vi "Init.vi"(10 "input":string[](array[string]), 11 "Volcano in":refnum<class "Volcano.lvclass">) -> (3 "Volcano out":refnum<class "Volcano.lvclass">)   [LabVIEW 2023, in "d16.lvlib" / "Volcano.lvclass"]
uses:
  Volcano.lvclass
  Volcano.lvclass/Volcano.ctl
  317e8209-662c-4c31-af41-99644d260e76.vi
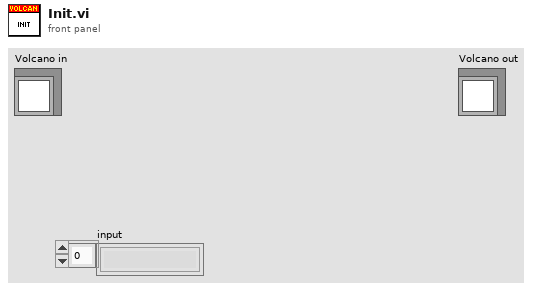
[diagram p1: front panel]
types:
  T1 = map{string, cluster{"Flow Rate":i32, "Routes":string[], "Route Time":i32[]}}
  T2 = cluster{"Current Valve":string, "Unopened Valves":string[], "Cumulative Pressure Released":u64, "Time":i32}
  T3 = cluster{"Flow Rate":i32, "Routes":string[], "Route Time":i32[]}
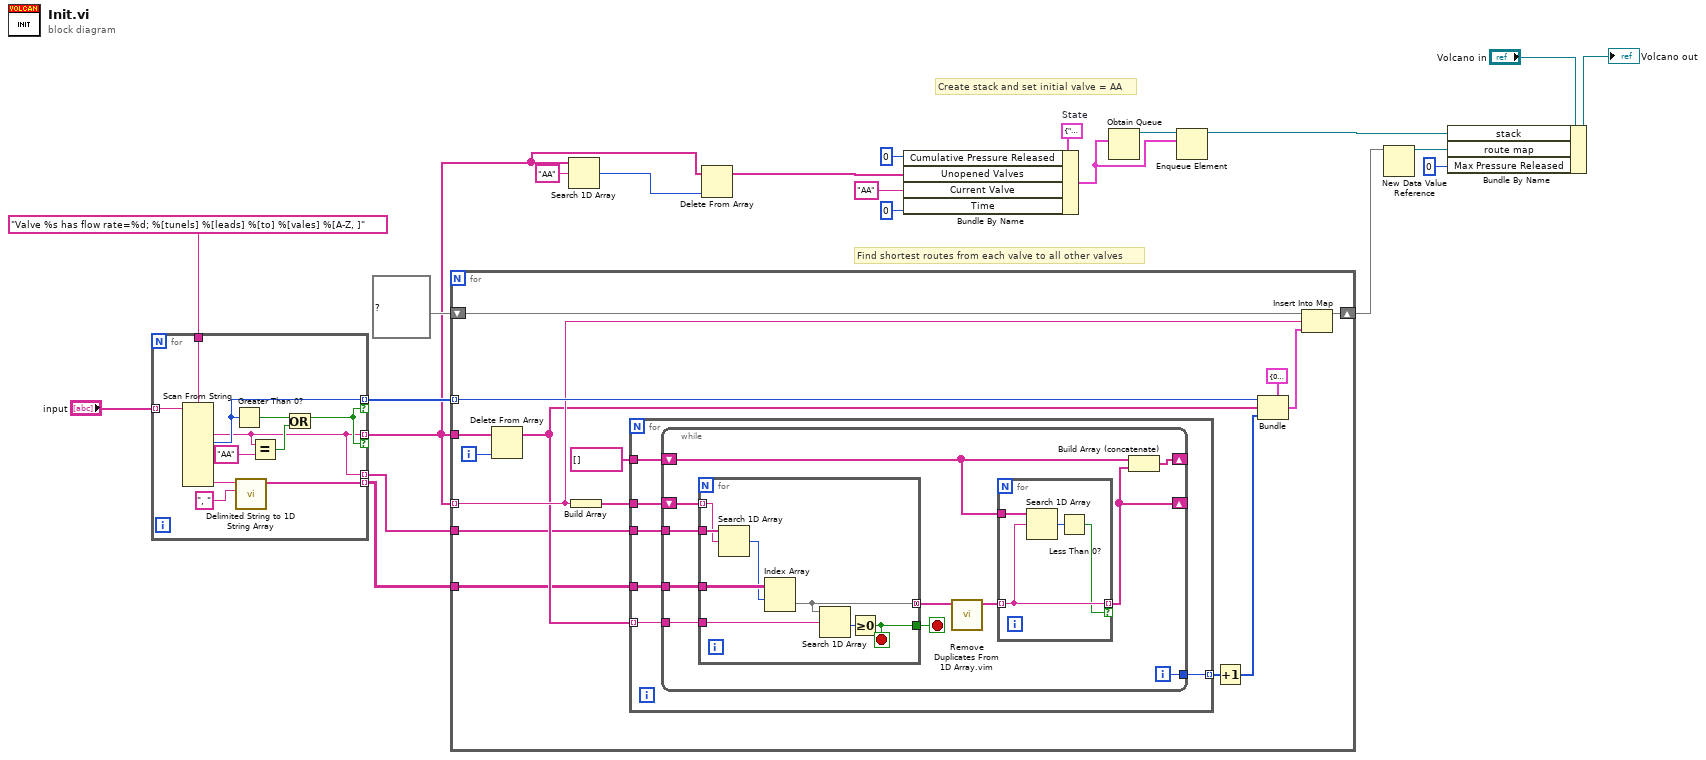
[diagram p0: block diagram]
diagram:
  w15 = T2 {"Current Valve"="AA", "Unopened Valves"=["AA"], "Cumulative Pressure Released"=0, "Time"=0}  # State
  # "Find shortest routes from each valve to all other valves"
  # "Create stack and set initial valve = AA"
  n1 = for {
    tunnel: "input" -> [w33] mode=indexing
    tunnel: "Valve %s has flow rate=%d; %[tunels] %[leads] %[to] %[vales] %[A-Z, ]" ("format string") -> [w32]
    tunnel: [w24] -> w2 mode=indexing if=w26
    tunnel: [w24] -> w20 mode=indexing
    tunnel: [w29] -> w19 mode=indexing if=w26
    tunnel: [w27] -> w18 mode=indexing
    n2 = Scan From String(format string=w32, input string=w33) -> (output 1=w24:string, output 2=w29:i32, output 7=w30:string)  [unwired: 13 in, 3 out]
    n3 = Greater Than 0?(x=w29) -> (x > 0?=w28:bool)
    n4 = call <vilib>:"Delimited String to 1D String Array.vi"("delimiter"=", ", "delimited string"=w30) -> ("string array"=w27:string[])  [unwired: 9 in]
    n5 = Equal?(x=w24, y="AA") -> (x = y?=w25:bool)
    n6 = Or(x=w28, y=w25) -> (x .or. y?=w26:bool)
  }
  n7 = for {
    tunnel: w20 -> [w40]
    tunnel: w2 -> [w42] mode=indexing
    tunnel: w2 -> [w46]
    shift-right: [w48] -> w7
    shift-left: T1 {} ("map out") -> [w47]
    tunnel: w19 -> [w44] mode=indexing
    tunnel: w18 -> [w39]
    i -> [w45]
    n8 = Delete From Array(array=w46, index=w45) -> (array with subset deleted=w41:string[])  [unwired: 1 in, 1 out]
    n9 = Build Array(w42) -> (w38:string[])
    n10 = for {
      tunnel: w41 -> [w54] mode=indexing
      tunnel: w40 -> [w53]
      tunnel: w39 -> [w52]
      tunnel: w38 -> [w51]
      tunnel: [w50] -> w37 mode=indexing
      tunnel: string[] [] -> [w49]
      n11 = while {
        tunnel: w54 -> [w63]
        tunnel: w53 -> [w65]
        shift-right: [w55] -> _
        shift-left: w51 -> [w60]
        tunnel: [w62] -> w50
        shift-right: [w56] -> _
        shift-left: w49 -> [w57]
        tunnel: w52 -> [w64]
        i -> [w62]
        stop <- w61 stop-if-true
        n12 = for {
          tunnel: w65 -> [w77]
          tunnel: w60 -> [w70] mode=indexing
          tunnel: w64 -> [w76]
          tunnel: [w74] -> w59 mode=concatenating
          tunnel: w63 -> [w73]
          tunnel: [w71] -> w61
          stop <- w71 stop-if-true
          n13 = Search 1D Array(1D array=w77, element=w70) -> (index of element=w75:i32)  [unwired: 1 in]
          n14 = Index Array(array=w76, index (row)=w75) -> (element=w74:string[])  [unwired: 1 in]
          n15 = Search 1D Array(1D array=w74, element=w73) -> (index of element=w72:i32)  [unwired: 1 in]
          n16 = Greater Or Equal To 0?(x=w72) -> (x >= 0?=w71:bool)
        }
        n17 = call "Remove Duplicates From 1D Array.vim"("array"=w59) -> ("array with duplicates removed"=w58:string[])  [unwired: 10 in]
        n18 = for {
          tunnel: w58 -> [w68] mode=indexing
          tunnel: w57 -> [w69]
          tunnel: [w68] -> w55 mode=indexing if=w66
          n19 = Search 1D Array(1D array=w69, element=w68) -> (index of element=w67:i32)  [unwired: 1 in]
          n20 = Less Than 0?(x=w67) -> (x < 0?=w66:bool)
        }
        n21 = Build Array (concatenate)(w57, w55) -> (w56:string[])
      }
    }
    n22 = Increment(x=w37) -> (x+1=w36:i32[])
    n23 = Bundle(cluster=T3 {"Flow Rate"=0, "Routes"=[], "Route Time"=[]}, "Flow Rate"=w44, "Routes"=w41, "Route Time"=w36) -> (w43:T3)
    n24 = Insert Into Map(map in=w47, key=w42, value=w43) -> (map out=w48:T1)  [unwired: 2 out]
  }
  n25 = Search 1D Array(1D array=w2, element="AA") -> (index of element=w1:i32)  [unwired: 1 in]
  n26 = Delete From Array(array=w2, index=w1) -> (array with subset deleted=w4:string[])  [unwired: 1 in, 1 out]
  n27 = Bundle By Name(cluster=w15, "Cumulative Pressure Released"=u64 0, "Unopened Valves"=w4, "Current Valve"="AA", "Time"=0) -> (w12:T2)
  n28 = Obtain Queue(element data type=w12) -> (queue out=w13:refnum<queue>)  [unwired: 4 in, 2 out]
  n29 = Enqueue Element(queue=w13, element=w12) -> (queue out=w5:refnum<queue>)  [unwired: 2 in, 2 out]
  n30 = New Data Value Reference(data value=w7) -> (data value reference=w10:refnum<data-value>)  [unwired: 1 in, 1 out]
  n31 = Bundle By Name(cluster="Volcano in", "stack"=w5, "route map"=w10, "Max Pressure Released"=u64 0) -> (→"Volcano out":refnum<class "Volcano.lvclass">)
